vi "WfLOfpaTester.vi"() -> ()   [LabVIEW 2013]
panel:
  in  "Delay (ms) In":i32=1000
  out "number (0 to 1)":dbl
  out "millisecond timer value":u32
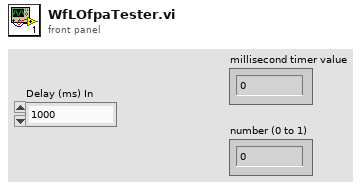
[diagram p1: front panel]
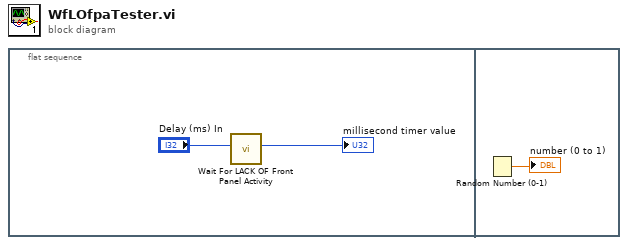
[diagram p0: block diagram]
diagram:
  n1 = flat-sequence {
    frame #0 {
      n2 = call "Wait For LACK OF Front Panel Activity.vi"("Delay (ms) In"="Delay (ms) In") -> ("Delay (ms) Out"=→"millisecond timer value":i32)  [unwired: 9 in]
    }
    frame #1 {
      n3 = Random Number (0-1)() -> (number: 0 to 1=→"number (0 to 1)":dbl)
    }
  }
